vi "Build Sensors.vi"(0 "Puzzle Input":string="Sensor at x=2, y=18: closest beacon is at x=-2, y=15\nSensor at x=9, y=16: closest beacon is at x=10, y=16\nSensor at x=13, y=2: closest beacon is at x=15, y=3\nSensor at x=12, y=14: closest beacon is at x=10, y=16\nSensor at x=10, y=20: closest beacon is at x=10, y=16\nSensor at x=14, y=17: closest beacon is at x=10, y=16\nSensor at x=8, y=7: closest beacon is at x=2, y=10\nSensor at x=2, y=0: closest beacon is at x=2, y=10\nSensor at x=0, y=11: closest beacon is at x=2, y=10\nSensor at x=20, y=14: closest beacon is at x=25, y=17\nSensor at x=17, y=20: closest beacon is at x=21, y=22\nSensor at x=16, y=7: closest beacon is at x=15, y=3\nSensor at x=14, y=3: closest beacon is at x=15, y=3\nSensor at x=20, y=1: closest beacon is at x=15, y=3") -> (1 "Boundary":T2, 2 "Sensors":map{T1, T3}(c390), 3 "Beacons":set{T1}(c389))   [LabVIEW 2020, in "AoC 2022.lvlib"]
uses:
  AoC 2022.lvlib
  Location.ctl
  Sensor Info.ctl
  Coverage Area.ctl
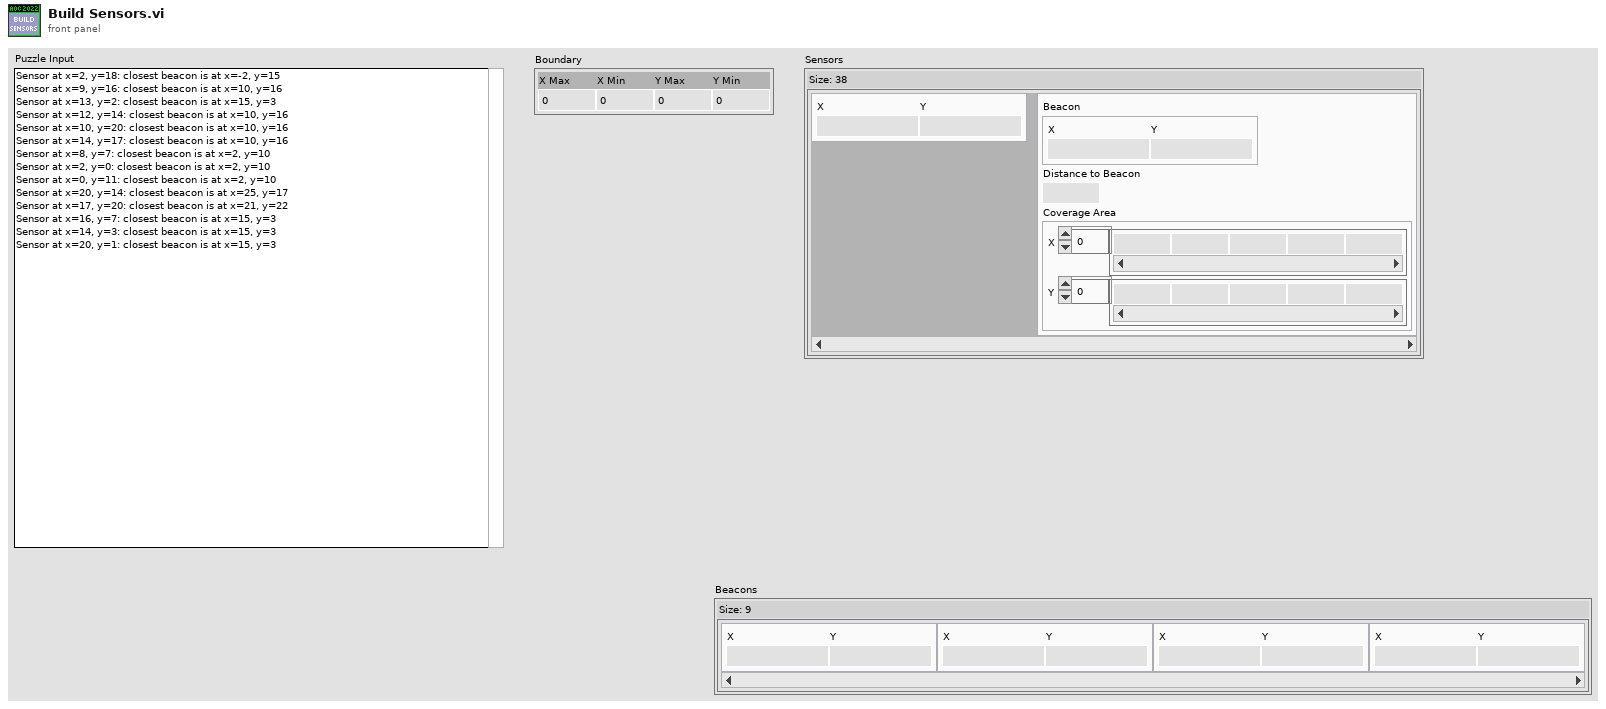
[diagram p1: front panel]
types:
  T1 = typedef "AoC 2022.lvlib/Location.ctl" = cluster{"X":i64, "Y":i64}
  T2 = cluster{"X Max":i32, "X Min":i32, "Y Max":i32, "Y Min":i32}
  T3 = typedef "AoC 2022.lvlib/Sensor Info.ctl" = cluster{"Beacon":T1, "Distance to Beacon":dbl, "Coverage Area":T4}
  T4 = typedef "AoC 2022.lvlib/Coverage Area.ctl" = cluster{"X":dbl[], "Y":dbl[]}
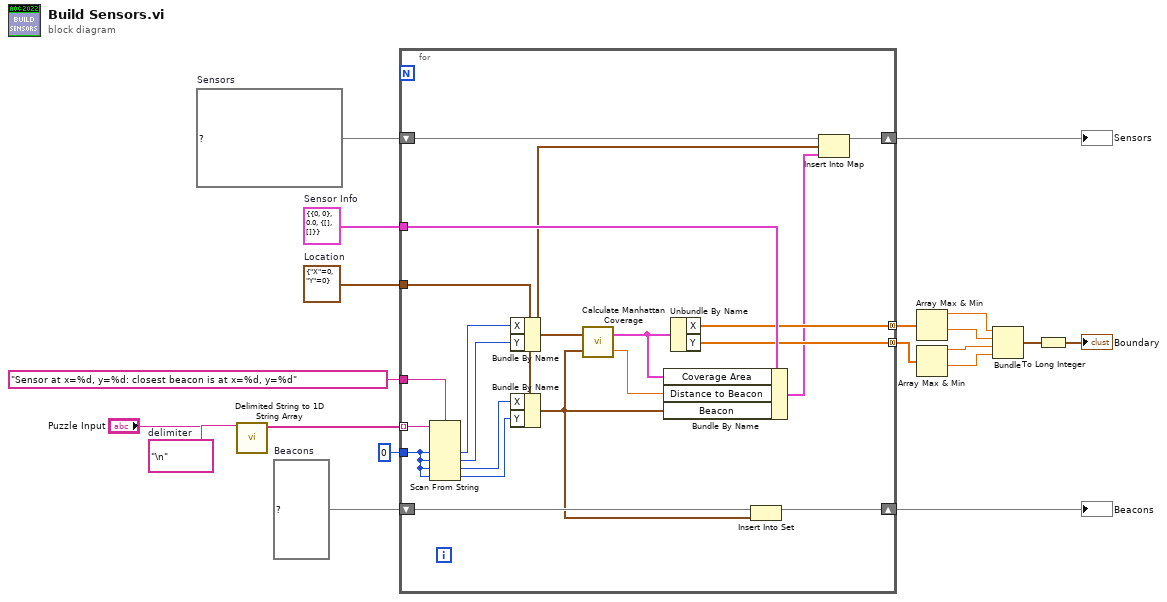
[diagram p0: block diagram]
diagram:
  w4 = "\n"  # delimiter
  w6 = set{T1} {}  # Beacons
  w16 = T3 {"Beacon"={"X"=0, "Y"=0}, "Distance to Beacon"=0.0, "Coverage Area"={"X"=[], "Y"=[]}}  # Sensor Info
  w15 = T1 {"X"=0, "Y"=0}  # Location
  w14 = map{T1, T3} {}  # Sensors
  n1 = call <vilib>:"Delimited String to 1D String Array.vi"("delimiter"=w4, "delimited string"="Puzzle Input") -> ("string array"=w2:string[])  [unwired: 9 in]
  n2 = for {
    tunnel: w2 -> [w39] mode=indexing
    tunnel: "Sensor at x=%d, y=%d: closest beacon is at x=%d, y=%d" -> [w38]
    shift-right: [w34] -> w19
    shift-left: w14 -> [w35]
    tunnel: w15 -> [w37]
    tunnel: w16 -> [w36]
    tunnel: [w27] -> w17 mode=concatenating
    tunnel: [w26] -> w18 mode=concatenating
    shift-right: [w22] -> w5
    shift-left: w6 -> [w23]
    tunnel: i64 0 -> [w20]
    n3 = Scan From String(format string=w38, input string=w39, default 1=w20, default 2=w20, default 3=w20, default 4=w20) -> (output 1=w30:i64, output 2=w31:i64, output 3=w29:i64, output 4=w32:i64)  [unwired: 2 in, 3 out]
    n4 = Bundle By Name(cluster=w37, "X"=w30, "Y"=w31) -> (w33:T1)
    n5 = Bundle By Name(cluster=w37, "X"=w29, "Y"=w32) -> (w21:T1)
    n6 = call "Calculate Manhattan Coverage.vi"("Destination"=w21, "Origin"=w33) -> ("Manhattan Distance"=w24:dbl, "Coverage Area"=w28:T4)
    n7 = Bundle By Name(cluster=w36, "Coverage Area"=w28, "Distance to Beacon"=w24, "Beacon"=w21) -> (w25:T3)
    n8 = Unbundle By Name(w28) -> ("X"=w27:dbl[], "Y"=w26:dbl[])
    n9 = Insert Into Set(10:w21, 11:w23) -> (3:w22:set{T1})  [unwired: 1 out]
    n10 = Insert Into Map(map in=w35, key=w33, value=w25) -> (map out=w34:map{T1, T3})  [unwired: 2 out]
  }
  "Sensors" <- w19
  "Beacons" <- w5
  n11 = Array Max & Min(array=w17) -> (max value=w12:dbl, min value=w11:dbl)  [unwired: 2 out]
  n12 = Array Max & Min(array=w18) -> (max value=w10:dbl, min value=w9:dbl)  [unwired: 2 out]
  n13 = Bundle(w12, w11, w10, w9) -> (w8:cluster{dbl, dbl, dbl, dbl})  [unwired: 1 in]
  n14 = To Long Integer(number=w8) -> (32bit integer=→"Boundary":cluster{i32, i32, i32, i32})
